vi "ConvertToCartesianVector.vi"(8 "error in (no error)":errorcluster, 11 "PolarVector in":refnum<class "PolarVector.lvclass">) -> (0 "error out":errorcluster, 3 "CartesianVector.lvclass":refnum<class "CartesianVector.lvclass">)   [LabVIEW 2011, in "PolarVector.lvclass"]
doc: "Converts a PolarVector class object to a CartesianVector class object."
uses:
  PolarVector.lvclass
  CartesianVector/CartesianVector.lvclass
  PolarVector.lvclass/PolarVector.ctl
  Angles/Angle/Angle.lvclass
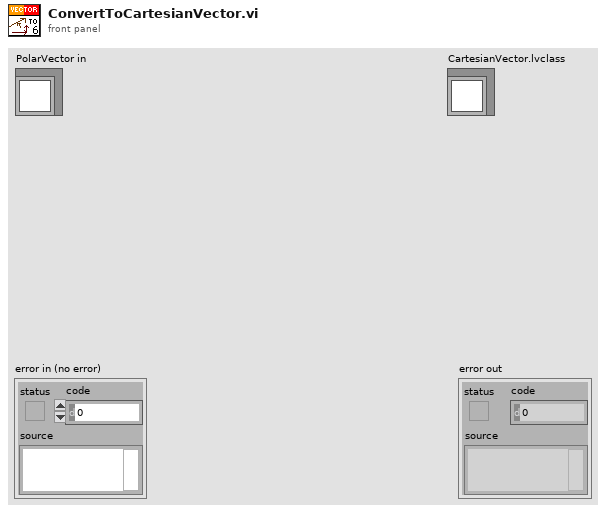
[diagram p1: front panel]
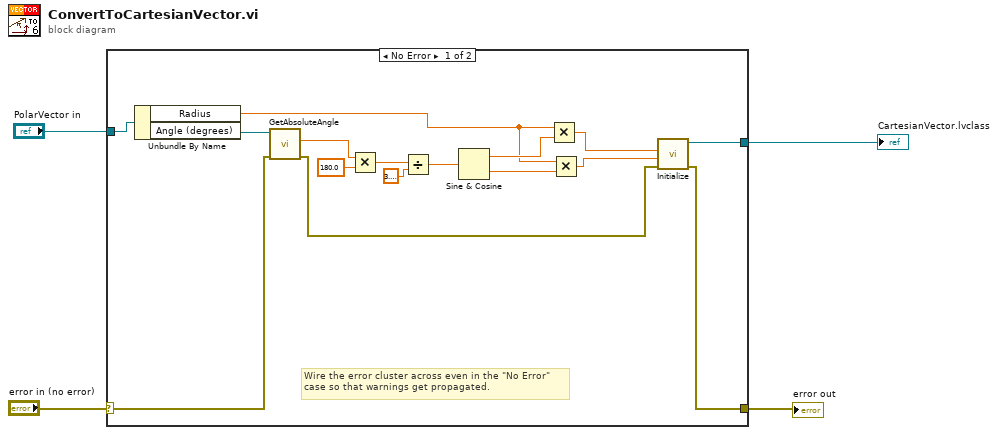
[diagram p0: block diagram]
diagram:
  n1 = case shown="No Error" "error in (no error)" {
    selector: "error in (no error)" -> [w11 w21]
    tunnel: [w6 w21] -> w2
    tunnel: "PolarVector in" -> [w14 _]
    tunnel: [w5 _] -> w1
    frame No Error {
      # "Wire the error cluster across even in the \"No Error\"\ncase so that warnings get propagated."
      n2 = Unbundle By Name(w14) -> ("Radius"=w10:dbl, "Angle (degrees)"=w13:refnum<class "Angle.lvclass">)
      n3 = call "GetAbsoluteAngle.vi"("error in (no error)"=w11, "Angle in"=w13) -> ("error out"=w7:errorcluster, "Absolute angle (Deg.)"=w12:dbl)  [unwired: 8 in]
      n4 = Multiply(x=w12, y=180.0) -> (x*y=w18:dbl)
      n5 = Divide(x=w18, y=3.141592653589793) -> (x/y=w17:dbl)
      n6 = Sine & Cosine(0:w17) -> (1:w15:dbl, 2:w20:dbl)
      n7 = Multiply(x=w10, y=w15) -> (x*y=w9:dbl)
      n8 = Multiply(x=w10, y=w20) -> (x*y=w8:dbl)
      n9 = call "Initialize.vi"("error in (no error)"=w7, "Y (North)"=w8, "X (East)"=w9) -> ("error out"=w6:errorcluster, "CartesianVector out"=w5:refnum<class "CartesianVector.lvclass">)  [unwired: 7 in]
    }
    frame Error {
    }
  }
  "error out" <- w2
  "CartesianVector.lvclass" <- w1
